vi "Impedance tube v0.3_complex_ratio.vi"() -> ()   [LabVIEW 2021]
uses:
  <vilib>/Analysis/2dsp.llb/Real FFT.vi
  <vilib>/express/express arith-compare/Formula/XNode/ExpressFormulaBlockNode.xnode
  <vilib>/Analysis/NI_AALPro.lvlib
panel:
  out "probe 1":dbl[](graph)
  out "Reflection coefficient":dbl[](graph)
  out "Absorption Coefficient":dbl[](graph)
  out "FFT {2}":cdb[](array[numeric])
  out "FFT {1}":cdb[](array[numeric])
  out "Transfer function":dbl[](graph)
  out "MIC 2":dynamicdata(graph)
  out "FFT2":dbl[](graph)
  in  "FFT size 2":i32=-1
  out "MIC 2":dbl
  out "FFT1":dbl[](graph)
  out "MIC 1":dynamicdata(graph)
  in  "FFT size":i32=-1
  out "MIC 1":dbl
  in  "stop (F)":bool
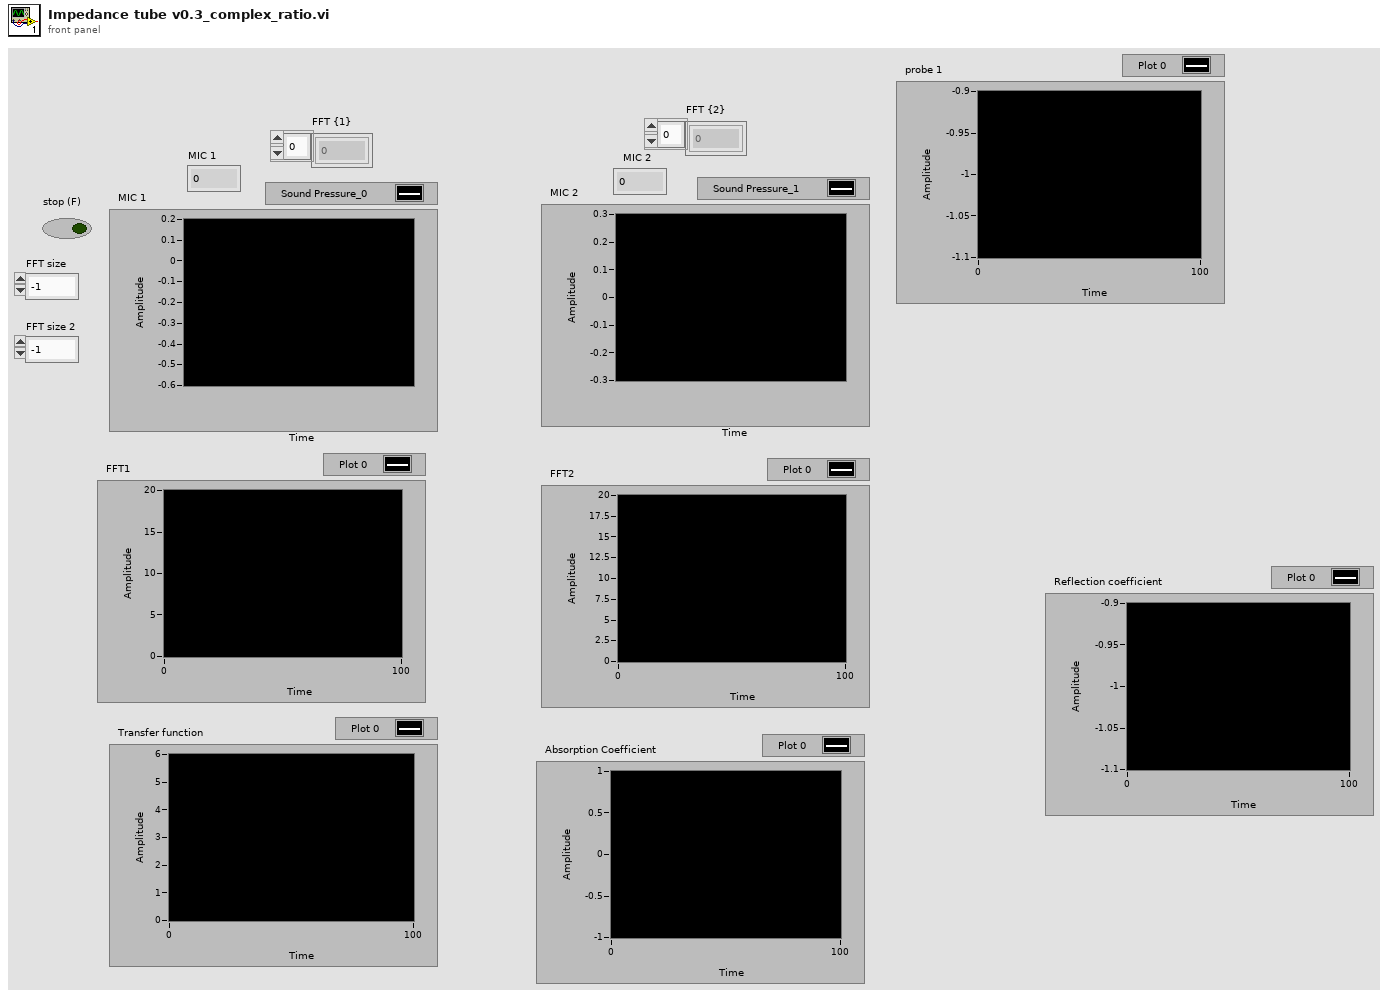
[diagram p1: front panel]
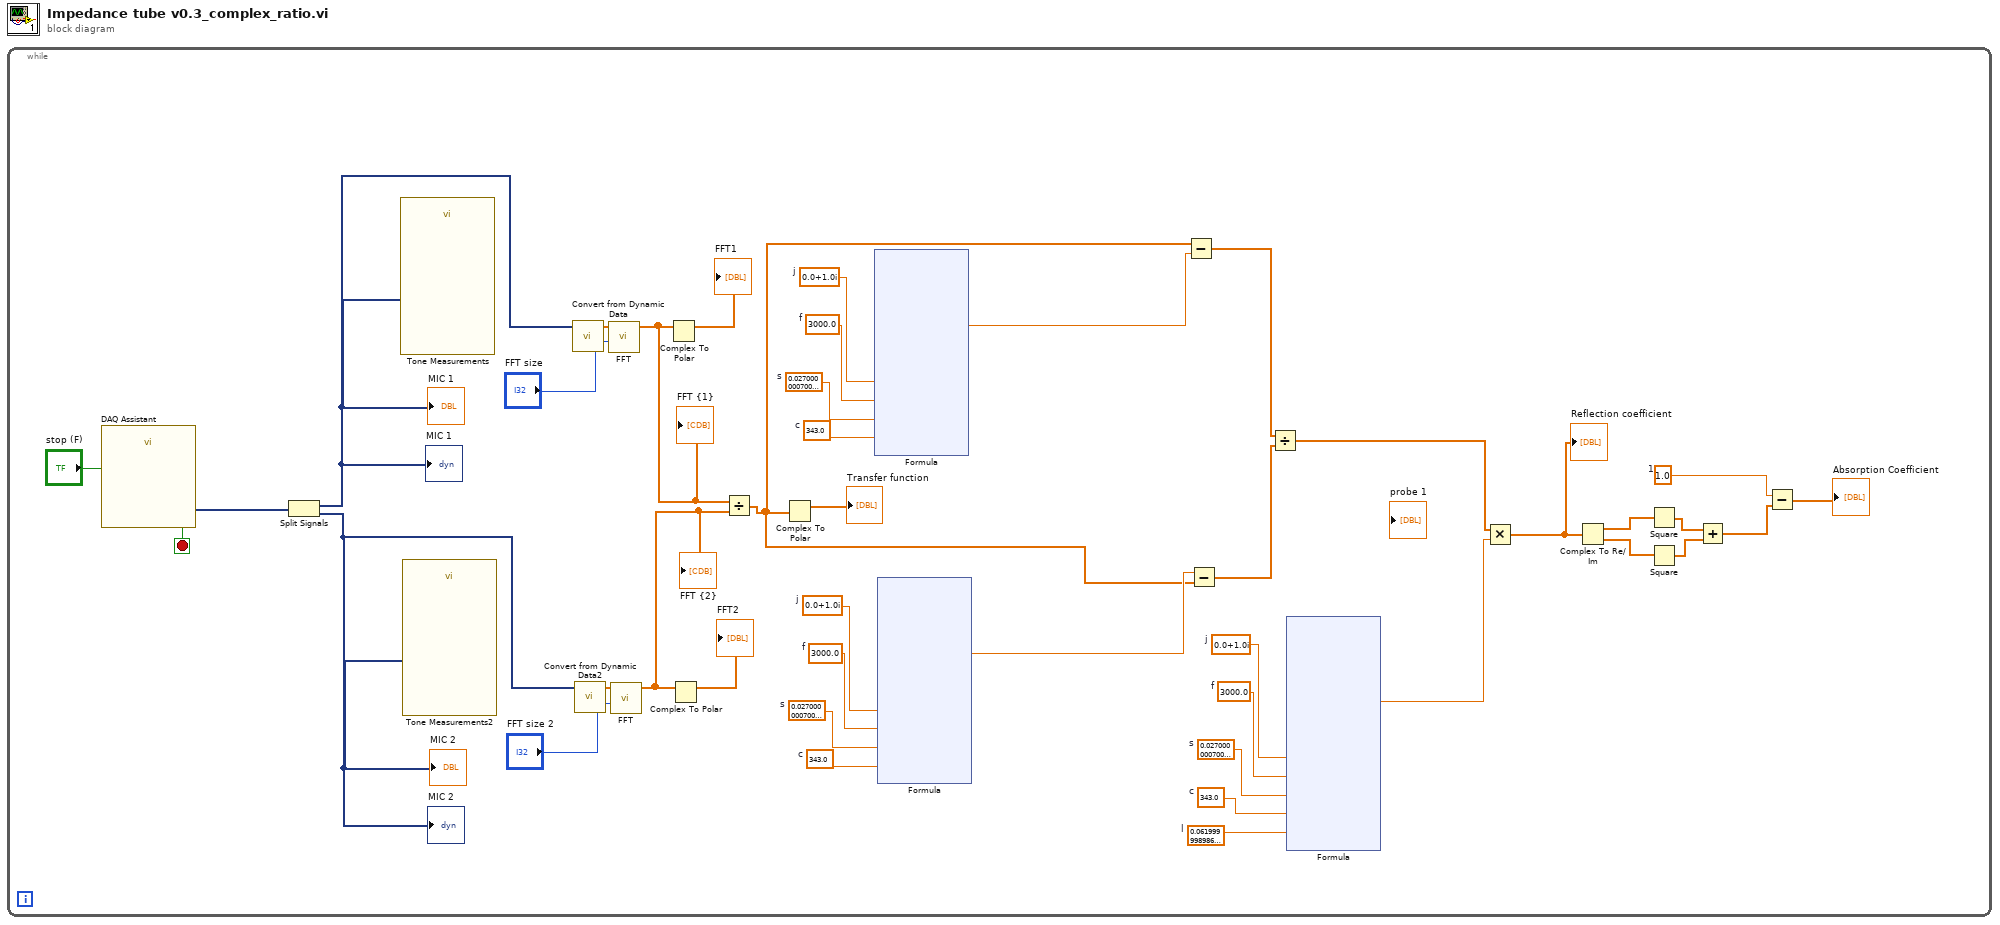
[diagram p0: block diagram]
diagram:
  n1 = while {
    stop <- w41 stop-if-true
    w8 = sgl 1.0  # 1
    w14 = sgl 0.062  # l
    w17 = sgl 3000.0  # f
    w16 = sgl 0.027  # s
    w15 = sgl 343.0  # c
    w18 = csg 0.0+1.0i  # j
    w22 = sgl 3000.0  # f
    w21 = sgl 0.027  # s
    w20 = sgl 343.0  # c
    w23 = csg 0.0+1.0i  # j
    w27 = sgl 3000.0  # f
    w26 = sgl 0.027  # s
    w25 = sgl 343.0  # c
    w28 = csg 0.0+1.0i  # j
    n2 = call "DAQ Assistant"("stop (F)"="stop (F)") -> ("data"=w37:dynamicdata, "stopped"=w41:bool)  [unwired: 15 in, 2 out]
    n3 = Split Signals(w37) -> (w33:dynamicdata, w30:dynamicdata)  [unwired: 2 in]
    "MIC 1" <- w33
    "MIC 1" <- w33
    "MIC 2" <- w30
    "MIC 2" <- w30
    n4 = call "Tone Measurements"("Signals"=w33) -> ()  [unwired: 8 in, 3 out]
    n5 = call "Tone Measurements2"("Signals"=w30) -> ()  [unwired: 8 in, 3 out]
    n6 = call "Convert from Dynamic Data"("Dynamic Data Type"=w33) -> ("Array"=w39:dbl[])  [unwired: 3 in]
    n7 = call "Convert from Dynamic Data2"("Dynamic Data Type"=w30) -> ("Array"=w35:dbl[])  [unwired: 3 in]
    n8 = call-poly <vilib>:"FFT.vi"("FFT size"="FFT size", "X"=w39) -> ("FFT {X}"=w32:cdb[])  [unwired: 8 in, 1 out]
    "FFT {1}" <- w32
    n9 = call-poly <vilib>:"FFT.vi"("FFT size"="FFT size 2", "X"=w35) -> ("FFT {X}"=w31:cdb[])  [unwired: 8 in, 1 out]
    "FFT {2}" <- w31
    n10 = Complex To Polar(r * e^(i*theta)=w32) -> (r=→"FFT1":dbl[])  [unwired: 1 out]
    n11 = Complex To Polar(r * e^(i*theta)=w31) -> (r=→"FFT2":dbl[])  [unwired: 1 out]
    n12 = Divide(x=w32, y=w31) -> (x/y=w4:cdb[])
    n13 = Complex To Polar(r * e^(i*theta)=w4) -> (r=→"Transfer function":dbl[])  [unwired: 1 out]
    n14 = xnode "Formula"("j"=w28, "f"=w27, "s"=w26, "c"=w25) -> ("Result"=w24:dbl)  [unwired: 1 in, 1 out]
    n15 = xnode "Formula"("j"=w23, "f"=w22, "s"=w21, "c"=w20) -> ("Result"=w19:dbl)  [unwired: 1 in, 1 out]
    n16 = Subtract(x=w4, y=w24) -> (x-y=w3:cdb[])
    n17 = Subtract(x=w19, y=w4) -> (x-y=w2:cdb[])
    n18 = Divide(x=w3, y=w2) -> (x/y=w1:cdb[])
    n19 = xnode "Formula"("j"=w18, "f"=w17, "s"=w16, "c"=w15, "l"=w14) -> ("Result"=w13:dbl)  [unwired: 1 in, 1 out]
    n20 = Multiply(x=w1, y=w13) -> (x*y=w5:cdb[])
    "Reflection coefficient" <- w5
    n21 = Complex To Re/Im(x + iy=w5) -> (x=w12:dbl[], y=w11:dbl[])
    n22 = Square(x=w12) -> (x^2=w10:dbl[])
    n23 = Square(x=w11) -> (x^2=w9:dbl[])
    n24 = Add(x=w10, y=w9) -> (x+y=w7:dbl[])
    n25 = Subtract(x=w8, y=w7) -> (x-y=→"Absorption Coefficient":dbl[])
  }
